vi "Test Comm.vi"() -> ()   [LabVIEW 2021]
uses:
  CIFChannels/Typedef/Direction.ctl
  CIF_NIChn_Fifo_Power.lvclass
  ChannelCommon/typedef/FIFO Config.ctl
  ChannelCommon/typedef/Datatype Waveform.ctl
  ChannelCommon/typedef/TimeStamps.ctl
  <vilib>/CIF Foundation/CIF Utilities/DataTypes/Flatten U64.vi
  ChannelCommon/ChannelCommon.lvlib
  CIFChannels/CIFChannels.lvclass
panel:
  out "status":string
  out "pass":bool
  out "error out":errorcluster
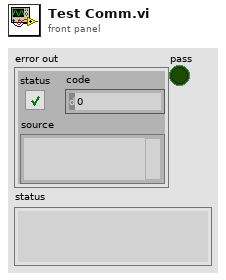
[diagram p1: front panel]
types:
  T1 = typedef "CIFChannels.lvclass/Direction.ctl" = enum16{"Publisher", "Subscriber"}
  T2 = typedef "ChannelCommon.lvlib/TimeStamps.ctl" = cluster{"ClockID":u8, "T0":i64, "T_Out":i64}
  T3 = typedef "ChannelCommon.lvlib/FIFO Config.ctl" = cluster{"Depth":u64, "Flags":u64}
  T4 = typedef "ChannelCommon.lvlib/Datatype Waveform.ctl" = cluster{"measurement":dbl[], "dT":dbl, "Timestamp":i64, "Read Lock":bool}
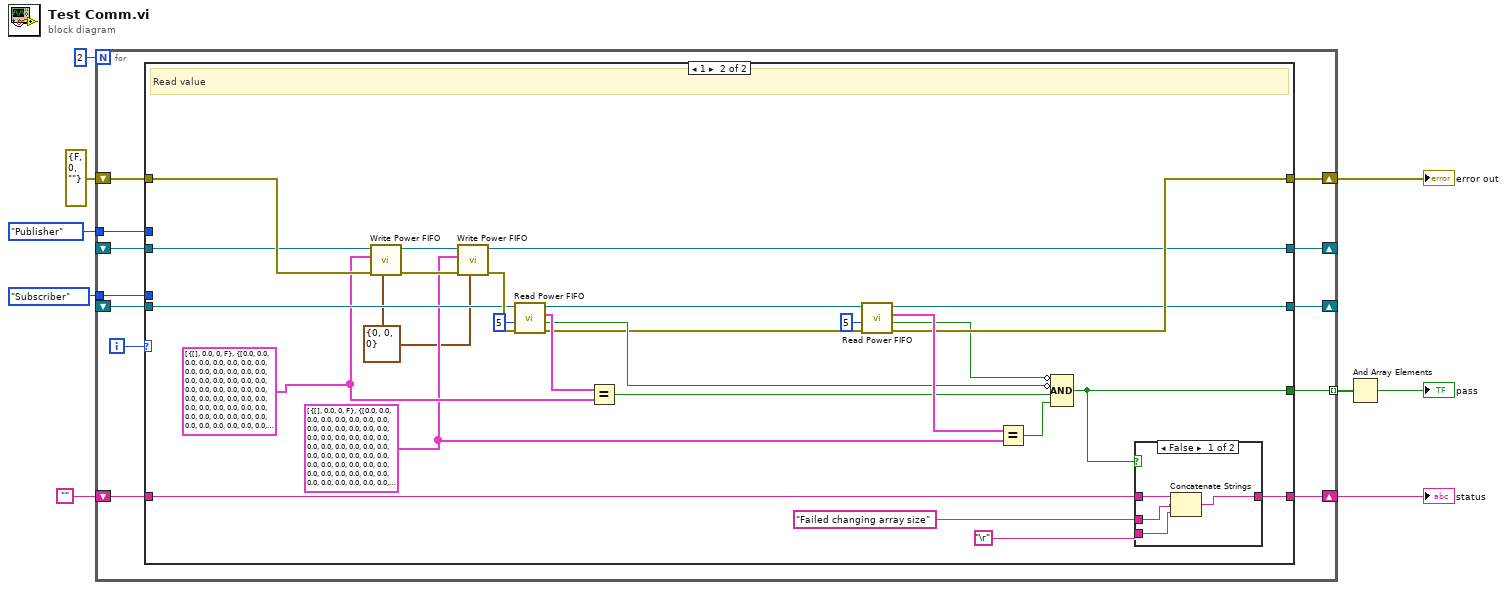
[diagram p0: block diagram]
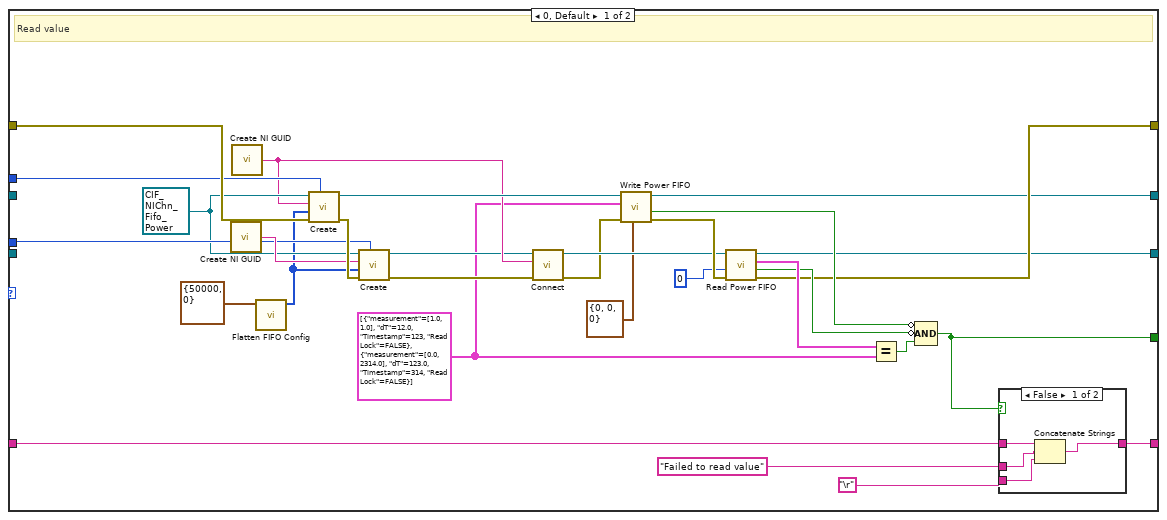
[diagram p2: hidden frame]
diagram:
  n1 = for {
    N: 2 -> [_]
    tunnel: [w21] -> w9 mode=indexing
    shift-right: [w19] -> w4
    shift-left: errorcluster {"status"=FALSE, "code"=0, "source"=""} ("error out") -> [w20]
    shift-right: [w16] -> w5
    shift-left: "" -> [w17]
    tunnel: Direction."Subscriber" ("Direction") -> [w15]
    tunnel: Direction."Publisher" ("Direction") -> [w14]
    shift-right: [w13] -> _
    shift-left: _ -> [w11]
    shift-right: [w12] -> _
    shift-left: _ -> [w10]
    i -> [w18]
    n2 = case shown="1" w18 {
      tunnel: [w46 w78] -> w21
      tunnel: w20 -> [w44 w72]
      tunnel: [w28 w76] -> w19
      tunnel: w17 -> [w51 w82]
      tunnel: [w50 w81] -> w16
      tunnel: w15 -> [w42 _]
      tunnel: w14 -> [w41 _]
      tunnel: [w26 w75] -> w13
      tunnel: [w25 w74] -> w12
      tunnel: w10 -> [_ w58]
      tunnel: w11 -> [_ w61]
      frame 0, Default {
        w24 = T4[] [{"measurement"=[1.0, 1.0], "dT"=12.0, "Timestamp"=123, "Read Lock"=FALSE}, {"measurement"=[0.0, 2314.0], "dT"=123.0, "Timestamp"=314, "Read Lock"=FALSE}] ("Data In")
        w40 = refnum<class "CIF_NIChn_Fifo_Power.lvclass"> refnum ("CIF_NIChn_Fifo_Power.lvclass")
        # "Read value"
        n3 = call <vilib>:"Create NI GUID.vi"() -> ("NI GUID"=w43:string)
        n4 = call <vilib>:"Create NI GUID.vi"() -> ("NI GUID"=w32:string)
        n5 = call "Flatten FIFO Config.vi"("FIFO Config in"=T3 {"Depth"=50000, "Flags"=0}) -> ("Flattened Data out"=w22:u8[])  [unwired: 10 in]
        n6 = call-dynamic "Create.vi"("Direction"=w41, "error in (no error)"=w44, "Custom Config Data"=w22, "Name"=w32, "CIFTag in"=w40) -> ("error out"=w45:errorcluster, "CIFTag out"=w38:refnum<class "CIF_NIChn_Fifo_Power.lvclass">)  [unwired: 5 in]
        n7 = call-dynamic "Create.vi"("Direction"=w42, "error in (no error)"=w45, "Custom Config Data"=w22, "Name"=w43, "CIFTag in"=w40) -> ("error out"=w31:errorcluster, "CIFTag out"=w29:refnum<class "CIF_NIChn_Fifo_Power.lvclass">)  [unwired: 5 in]
        n8 = call-dynamic "Connect.vi"("error in (no error)"=w31, "Connection Name"=w32, "CIFTag in"=w29) -> ("error out"=w30:errorcluster, "CIFTag out"=w33:refnum<class "CIF_NIChn_Fifo_Power.lvclass">)  [unwired: 7 in]
        n9 = call-dynamic "Write Power FIFO.vi"("FIFO Timestamps"=T2 {"ClockID"=0, "T0"=0, "T_Out"=0}, "error in (no error)"=w30, "Data In"=w24, "CIFTag in"=w38) -> ("error out"=w37:errorcluster, "timed out?"=w35:bool, "CIFTag out"=w25:refnum<class "CIF_NIChn_Fifo_Power.lvclass">)  [unwired: 4 in, 1 out]
        n10 = call-dynamic "Read Power FIFO.vi"("error in (no error)"=w37, "Timeout (ms)"=0, "CIFTag in"=w33) -> ("error out"=w28:errorcluster, "timed out?"=w34:bool, "Data out"=w36:T4[], "CIFTag out"=w26:refnum<class "CIF_NIChn_Fifo_Power.lvclass">)  [unwired: 4 in, 1 out]
        n11 = Equal?(x=w36, y=w24) -> (x = y?=w47:bool)
        n12 = Compound Arithmetic op=AND(invert w35, invert w34, w47) -> (w46:bool)
        n13 = case shown="False" w46 {
          tunnel: w51 -> [w55 w56]
          tunnel: [w52 w56] -> w50
          tunnel: "Failed to read value" -> [w54 _]
          tunnel: "\r" -> [w53 _]
          frame False {
            n14 = Concatenate Strings(w55, w54, w53) -> (w52:string)
          }
          frame True {
          }
        }
      }
      frame 1 {
        w57 = T2 {"ClockID"=0, "T0"=0, "T_Out"=0} ("FIFO Timestamps")
        w59 = T4[] [{"measurement"=[], "dT"=0.0, "Timestamp"=0, "Read Lock"=FALSE}, {"measurement"=[0.0, 0.0, 0.0, 0.0, 0.0, 0.0, 0.0, 0.0, 0.0, 0.0, 0.0, 0.0, 0.0, 0.0, 0.0, 0.0, 0.0, 0.0, 0.0, 0.0, 0.0, 0.0, 0.0, 0.0, 0.0, 0.0, 0.0, 0.0, 0.0, 0.0, 0.0, 0.0, 0.0, 0.0, 0.0, 0.0, 0.0, 0.0, 0.0, 0.0, 0.0, 0.0, 0.0, 0.0, 0.0, 0.0, 0.0, 0.0, 0.0, 0.0, 3.14, 0.0, 0.0, 0.0, 0.0, 0.0, 0.0, 0.0, 0.0, 0.0, 0.0, 0.0, 0.0, 0.0, 0.0, 0.0, 0.0, 0.0, 0.0, 0.0, 0.0, 0.0, 0.0, 0.0, 0.0, 0.0, 0.0, 0.0, 0.0, 0.0, 0.0, 0.0, 0.0, 0.0, 0.0, 0.0, 0.0, 0.0, 0.0, 0.0, 0.0, 0.0, 0.0, 0.0, 0.0, 0.0, 0.0, 0.0, 0.0, 0.0, 3.14], "dT"=5.2, "Timestamp"=523, "Read Lock"=FALSE}] ("Data In")
        w60 = T4[] [{"measurement"=[], "dT"=0.0, "Timestamp"=0, "Read Lock"=FALSE}, {"measurement"=[0.0, 0.0, 0.0, 0.0, 0.0, 0.0, 0.0, 0.0, 0.0, 0.0, 0.0, 0.0, 0.0, 0.0, 0.0, 0.0, 0.0, 0.0, 0.0, 0.0, 0.0, 0.0, 0.0, 0.0, 0.0, 0.0, 0.0, 0.0, 0.0, 0.0, 0.0, 0.0, 0.0, 0.0, 0.0, 0.0, 0.0, 0.0, 0.0, 0.0, 0.0, 0.0, 0.0, 0.0, 0.0, 0.0, 0.0, 0.0, 0.0, 0.0, 3.14], "dT"=5.2, "Timestamp"=523, "Read Lock"=FALSE}] ("Data In")
        # "Read value"
        n15 = call-dynamic "Write Power FIFO.vi"("FIFO Timestamps"=w57, "error in (no error)"=w72, "Data In"=w60, "CIFTag in"=w58) -> ("error out"=w66:errorcluster, "CIFTag out"=w73:refnum<class "CIF_NIChn_Fifo_Power.lvclass">)  [unwired: 4 in, 2 out]
        n16 = call-dynamic "Write Power FIFO.vi"("FIFO Timestamps"=w57, "error in (no error)"=w66, "Data In"=w59, "CIFTag in"=w73) -> ("CIFTag out"=w74:refnum<class "CIF_NIChn_Fifo_Power.lvclass">)  [unwired: 4 in, 3 out]
        n17 = call-dynamic "Read Power FIFO.vi"("error in (no error)"=w66, "Timeout (ms)"=5, "CIFTag in"=w61) -> ("error out"=w65:errorcluster, "timed out?"=w67:bool, "Data out"=w71:T4[], "CIFTag out"=w64:refnum<class "CIF_NIChn_Fifo_Power.lvclass">)  [unwired: 4 in, 1 out]
        n18 = Equal?(x=w71, y=w60) -> (x = y?=w69:bool)
        n19 = call-dynamic "Read Power FIFO.vi"("error in (no error)"=w65, "Timeout (ms)"=5, "CIFTag in"=w64) -> ("error out"=w76:errorcluster, "timed out?"=w68:bool, "Data out"=w77:T4[], "CIFTag out"=w75:refnum<class "CIF_NIChn_Fifo_Power.lvclass">)  [unwired: 4 in, 1 out]
        n20 = Equal?(x=w77, y=w59) -> (x = y?=w70:bool)
        n21 = Compound Arithmetic op=AND(invert w68, invert w67, w69, w70) -> (w78:bool)
        n22 = case shown="False" w78 {
          tunnel: w82 -> [w86 w87]
          tunnel: [w83 w87] -> w81
          tunnel: "Failed changing array size" -> [w85 _]
          tunnel: "\r" -> [w84 _]
          frame False {
            n23 = Concatenate Strings(w86, w85, w84) -> (w83:string)
          }
          frame True {
          }
        }
      }
    }
  }
  "error out" <- w4
  "status" <- w5
  n24 = And Array Elements(Boolean array=w9) -> (logical AND=→"pass":bool)
